vi "HW3.vi"() -> ()   [LabVIEW 2011]
panel:
  out "Lower":bool
  out "Close to":bool
  out "Higher":bool
  out "Temperature Chart":dbl(graph)
  in  "Take Data Point":bool caption="Sleeping"
  out "The Time":string
  in  "stop":bool
  out "Warning Light":u32(colorbox) caption="All Clear"
  out "Units":string
  in  "Unit Selector":u16(ring) items=["Celsius", "Fahrenheit", "Kelvin"]
  in  "Voltage":dbl(knob) scale=0.0..4.0 scale format="%#.3f"
  out "Temperature":dbl(knob) min=-400.0 max=550.0 scale=-400.0..550.0 scale format="%#.3g"
  # "Daniel Payne\nHW 2"
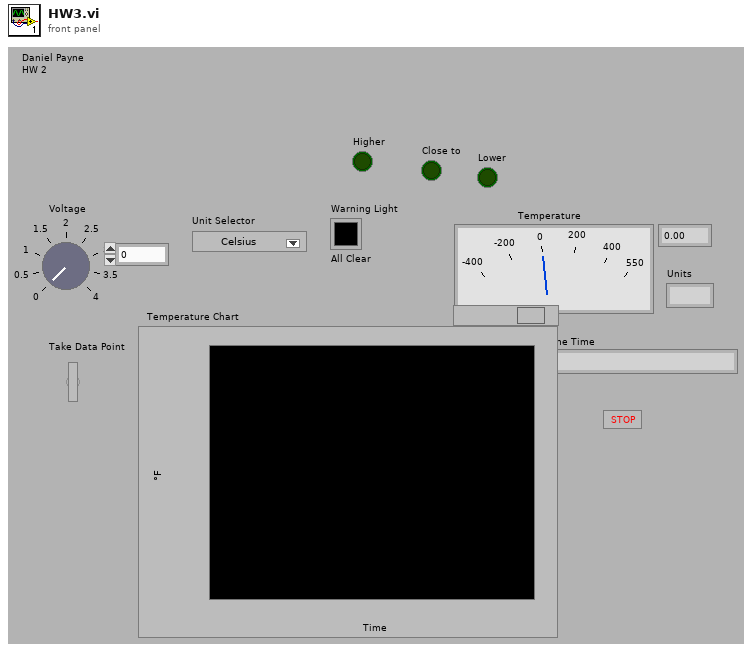
[diagram p1: front panel]
types:
  T1 = enum8{"Enabled", "Disabled", "Disabled and Grayed Out"}
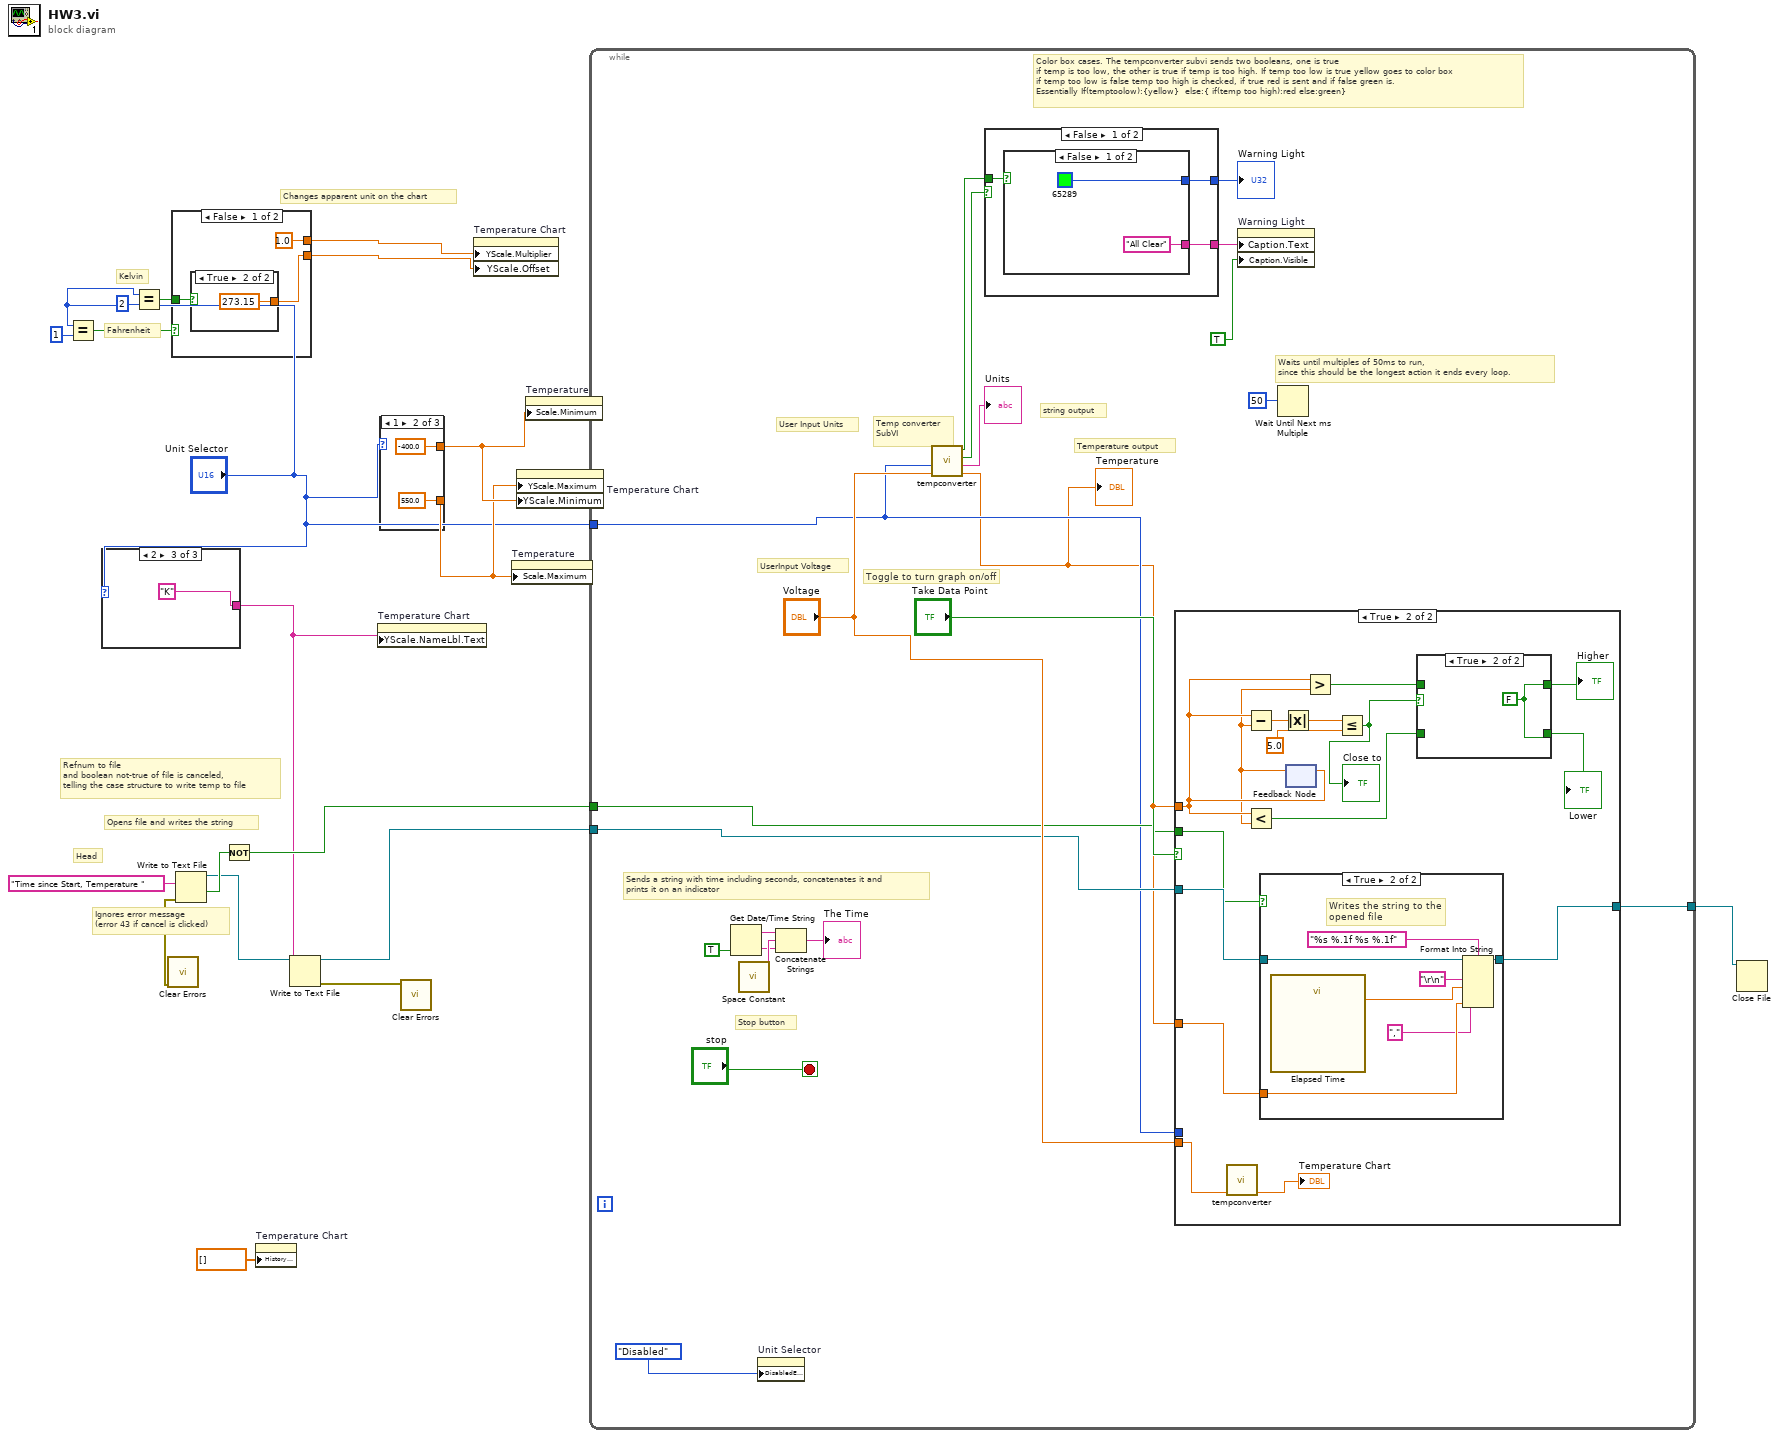
[diagram p0: block diagram]
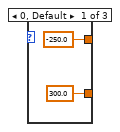
[diagram p2: hidden frame]
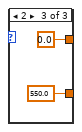
[diagram p3: hidden frame]
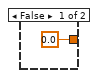
[diagram p4: hidden frame]
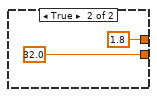
[diagram p5: hidden frame]
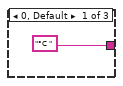
[diagram p6: hidden frame]
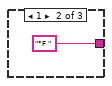
[diagram p7: hidden frame]
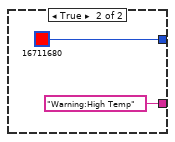
[diagram p11: hidden frame]
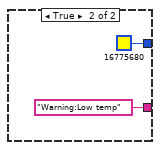
[diagram p12: hidden frame]
diagram:
  # "Changes apparent unit on the chart"
  # "Fahrenheit"
  # "Kelvin"
  # "Refnum to file \nand boolean not-true of file is canceled,\ntelling the case structure to write temp to file"
  # "Ignores error message\n(error 43 if cancel is clicked)"
  # "Opens file and writes the string"
  # "Head"
  n1 = Equal?(x="Unit Selector", y=1) -> (x = y?=w11:bool)
  n2 = case shown="2" "Unit Selector" {
    tunnel: ["°C " ("text") "°F " ("text") "K" ("text")] -> w7
    frame 0, Default {
    }
    frame 1 {
    }
    frame 2 {
    }
  }
  n3 = Equal?(x="Unit Selector", y=2) -> (x = y?=w10:bool)
  n4 = case shown="False" w11 {
    tunnel: w10 -> [w25 _]
    tunnel: [w24 32.0 ("X Scale.Offset and Multiplier:Multiplier")] -> w8
    tunnel: [1.0 ("X Scale.Offset and Multiplier:Offset") 1.8 ("X Scale.Offset and Multiplier:Multiplier")] -> w9
    frame False {
      n5 = case shown="True" w25 {
        tunnel: [0.0 ("X Scale.Offset and Multiplier:Offset") 273.15 ("X Scale.Offset and Multiplier:Offset")] -> w24
        frame False {
        }
        frame True {
        }
      }
    }
    frame True {
    }
  }
  n6 = Write to Text File(text="Time since Start, Temperature ") -> (refnum out=w15:refnum<file>, cancelled=w17:bool, error out=w6:errorcluster)  [unwired: 3 in]
  n7 = call <vilib>:"Clear Errors.vi"("error in (no error)"=w6) -> ()  [unwired: 6 in, 1 out]
  n8 = Not(x=w17) -> (.not. x?=w16:bool)
  n9 = property on="Temperature Chart" class="WFChart (strict)"("History Data"=dbl[] []) -> ()  [unwired: 2 in, 2 out]
  n10 = Write to Text File(file (use dialog)=w15, text=w7) -> (refnum out=w14:refnum<file>, error out=w5:errorcluster)  [unwired: 2 in, 1 out]
  n11 = property on="Temperature Chart" class="WFChart (strict)"("YScale.NameLbl.Text"=w7) -> ()  [unwired: 2 in, 2 out]
  n12 = case shown="1" "Unit Selector" {
    tunnel: [-250.0 ("Data Entry Limits:Maximum") -400.0 ("Data Entry Limits:Maximum") 0.0 ("Data Entry Limits:Maximum")] -> w4
    tunnel: [300.0 ("Data Entry Limits:Maximum") 550.0 ("Data Entry Limits:Maximum") 550.0 ("Data Entry Limits:Maximum")] -> w3
    frame 0, Default {
    }
    frame 1 {
    }
    frame 2 {
    }
  }
  n13 = call <vilib>:"Clear Errors.vi"("error in (no error)"=w5) -> ()  [unwired: 6 in, 1 out]
  n14 = property on="Temperature Chart" class="WFChart (strict)"("YScale.Multiplier"=w9, "YScale.Offset"=w8) -> ()  [unwired: 2 in, 2 out]
  n15 = property on="Temperature" class="Knob (strict)"("Scale.Maximum"=w3) -> ()  [unwired: 2 in, 2 out]
  n16 = property on="Temperature Chart" class="WFChart (strict)"("YScale.Maximum"=w3, "YScale.Minimum"=w4) -> ()  [unwired: 2 in, 2 out]
  n17 = property on="Temperature" class="Knob (strict)"("Scale.Minimum"=w4) -> ()  [unwired: 2 in, 2 out]
  n18 = while {
    tunnel: w16 -> [w42]
    tunnel: w14 -> [w40]
    tunnel: "Unit Selector" -> [w39]
    tunnel: [w37] -> w1
    stop <- "stop" stop-if-true
    # "Stop button"
    # "Toggle to turn graph on/off"
    # "Sends a string with time including seconds, concatenates it and\nprints it on an indicator"
    # "Waits until multiples of 50ms to run, \nsince this should be the longest action it ends every loop."
    # "Color box cases. The tempconverter subvi sends two booleans, one is true\nif temp is too low, the other is true if temp is too high. If temp too low is true yellow goes to color box\nif temp too low is false temp too high is checked, if true red is sent and if false green is.\nEssentially If(temptoolow):{yellow}  else:{ if(temp too high):red else:green}"
    # "string output"
    # "Temperature output"
    # "Temp converter\nSubVI"
    # "User Input Units"
    # "UserInput Voltage"
    n19 = Get Date/Time String(want seconds? (F)=TRUE) -> (date string=w50:string, time string=w48:string)  [unwired: 2 in]
    n20 = call <vilib>:"Space Constant.vi"() -> ("String"=w49:string)
    n21 = property on="Unit Selector" class="Ring (strict)"("DisabledEnum"=T1."Disabled" ("Disabled")) -> ()  [unwired: 2 in, 2 out]
    n22 = Concatenate Strings(w50, w49, w48) -> (→"The Time":string)
    n23 = call "tempconverter.vi"("Voltage"="Voltage", "Unit Selector"=w39) -> ("Temperature"=w36:dbl, "Units"=→"Units":string, "Input too low"=w56:bool, "Input too high"=w55:bool)  [unwired: 5 in]
    "Temperature" <- w36
    n24 = case shown="False" w56 {
      tunnel: w55 -> [w87 _]
      tunnel: [w86 u32 16775680 ("B")] -> w54
      tunnel: [w85 "Warning:Low temp"] -> w45
      frame False {
        n25 = case shown="False" w87 {
          tunnel: [u32 65289 ("B") u32 16711680 ("B")] -> w86
          tunnel: ["All Clear" "Warning:High Temp"] -> w85
          frame False {
          }
          frame True {
          }
        }
      }
      frame True {
      }
    }
    "Warning Light" <- w54
    n26 = case shown="True" "Take Data Point" {
      tunnel: w40 -> [w57 w73]
      tunnel: w42 -> [_ w72]
      tunnel: w39 -> [_ _]
      tunnel: w36 -> [_ w71]
      tunnel: "Voltage" -> [_ w70]
      tunnel: [w57 w68] -> w37
      tunnel: w36 -> [_ w64]
      frame False {
      }
      frame True {
        n27 = call "tempconverter.vi"("Voltage"=w70) -> ("Temperature"=→"Temperature Chart":dbl)  [unwired: 6 in, 3 out]
        n28 = case shown="True" w72 {
          tunnel: w73 -> [w77 w84]
          tunnel: w71 -> [_ w80]
          tunnel: [w77 w78] -> w68
          frame False {
          }
          frame True {
            # "Writes the string to the \nopened file"
            n29 = call "Elapsed Time"() -> ("Elapsed Time (s)"=w82:dbl)  [unwired: 12 in, 7 out]
            n30 = Format Into String(format string="%s %.1f %s %.1f", initial string=w84, "\r\n", w82, ",", w80) -> (resulting string=w78:refnum<file>)  [unwired: 1 in, 1 out]
          }
        }
        n31 = feedback-in #1(w64) -> ()
        n32 = feedback #1() -> (w63:dbl)  [unwired: 1 in]
        n33 = Subtract(x=w64, y=w63) -> (x-y=w66:dbl)
        n34 = Less?(x=w64, y=w63) -> (x < y?=w61:bool)
        n35 = Absolute Value(x=w66) -> (abs(x)=w67:dbl)
        n36 = Greater?(x=w64, y=w63) -> (0:w59:bool)
        n37 = Less Or Equal?(x=w67, y=5.0 ("x")) -> (x <= y?=w62:bool)
        "Close to" <- w62
        n38 = case shown="True" w62 {
          tunnel: [w75 w76] -> w60
          tunnel: w61 -> [w75 _]
          tunnel: w59 -> [w74 _]
          tunnel: [w74 w76] -> w58
          frame False {
          }
          frame True {
            w76 = FALSE
          }
        }
        "Higher" <- w58
        "Lower" <- w60
      }
    }
    n39 = property on="Warning Light" class="ColBox"("Caption.Text"=w45, "Caption.Visible"=TRUE) -> ()  [unwired: 2 in, 2 out]
    n40 = Wait Until Next ms Multiple(millisecond multiple=u32 50 ("milliseconds to wait")) -> ()  [unwired: 1 out]
  }
  n41 = Close File(refnum=w1) -> ()  [unwired: 1 in, 2 out]
